vi "Send Message.vi"(8 "error in (no error)":errorcluster, 10 "Message":string, 11 "WebSocket Client in":refnum<class "WebSocket Client.lvclass">) -> (0 "error out":errorcluster, 3 "WebSocket Client out":refnum<class "WebSocket Client.lvclass">)   [LabVIEW 2017, in "WebSocket Client.lvlib" / "WebSocket Client.lvclass"]
uses:
  WebSocket Client.lvclass
  WebSocket Client.lvclass/WebSocket Client.ctl
  <vilib>/MediaMongrels Ltd/WebSockets/Sockets/VISA TCP Socket/VISA TCP.lvclass
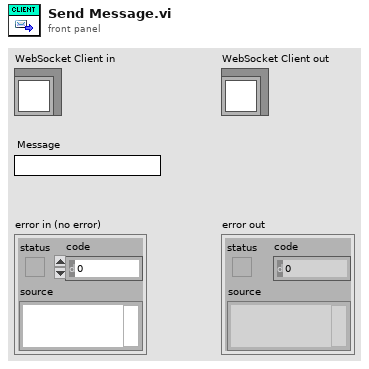
[diagram p1: front panel]
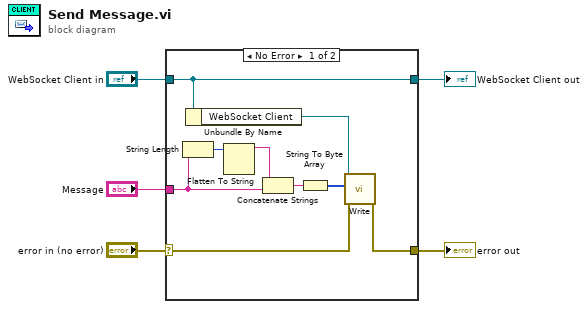
[diagram p0: block diagram]
diagram:
  n1 = case shown="No Error" "error in (no error)" {
    selector: "error in (no error)" -> [w12 w16]
    tunnel: [w11 w16] -> w4
    tunnel: [w14 w15] -> w2
    tunnel: "WebSocket Client in" -> [w14 w15]
    tunnel: "Message" -> [w7 _]
    frame No Error {
      n2 = String Length(string=w7) -> (length=w9:i32)
      n3 = Unbundle By Name(w14) -> ("WebSocket Client"=w13:refnum<class "VISA TCP.lvclass">)
      n4 = Flatten To String(anything=w9) -> (data string=w8:string)  [unwired: 1 in, 4 out]
      n5 = Concatenate Strings(w8, w7) -> (w6:string)
      n6 = String To Byte Array(string=w6) -> (unsigned byte array=w10:u8[])
      n7 = call-dynamic "Write.vi"("error in (no error)"=w12, "Bytes to write"=w10, "VISA TCP in"=w13) -> ("error out"=w11:errorcluster)  [unwired: 6 in, 2 out]
    }
    frame Error {
    }
  }
  "error out" <- w4
  "WebSocket Client out" <- w2
